vi "NI6071E.evt call DAQ Config.vi"(0 "i ref in":refnum<vi>, 2 "Client":string, 3 "Client timeout (10000)":i32=10000, 4 "NI6071E Config":T1={"device (1)"=1, "channels (0)"=[], "buffer size (1000 scans)"=1000, "[number of buffers] (1)"=1, "measurement mode structure"={"measurement mode"=0, "reserved"=0}, "input limits (no change)"=[], "coupling & input config (no change:0)"=[]} {"measurement mode structure"."measurement mode" items=["no change", "Volts", "Volts RMS", "Ohms", "Diode", "4-wire ohms", "Current", "Current RMS"]; "coupling & input config (no change:0)"."input config (no change:0)" items=["no change", "differential", "ref. single-ended", "non-ref. single-ended", "4-wire"]; "input limits (no change)"."low limit (0.0)" format="%0.2f"; "input limits (no change)"."high limit (0.0)" format="%0.2f"}, 5 "error in (no error)":errorcluster) -> (14 "i ref out":refnum<vi>, 19 "error out":errorcluster)   [LabVIEW 2014, in "NI6071E.lvlib"]
doc: "This VI asks for an event by a simple call"
uses:
  NI6071E.lvlib
  NI6071ECommand.ctl
  NI6071EConfig.ctl
  CSCore/CSSystem/CoreLib/CoreLib.string 2 byte array.vi
  CSCore/CSSystem/CoreLib/CoreLib.int 2 byte array.vi
  CSCore/BaseProcess/BaseProcess.lvlib
  CSCore/CSSystem/CoreLib/CoreLib.lvlib
panel:
  in  "NI6071E Command":T2=enum."ConfigureDAQ"
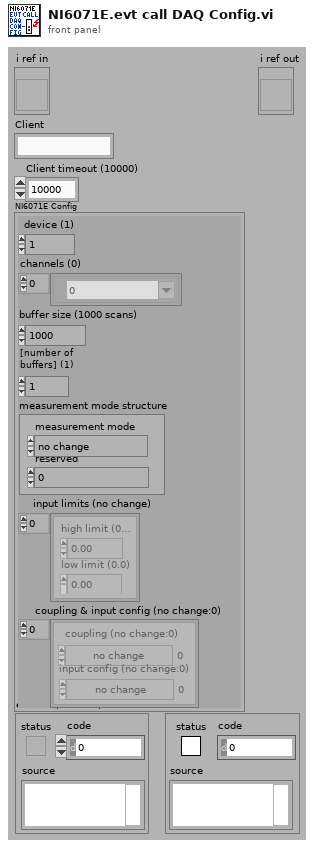
[diagram p1: front panel]
types:
  T1 = typedef "NI6071E.lvlib/NI6071EConfig.ctl" = cluster{"device (1)":i16, "channels (0)":tag[], "buffer size (1000 scans)":i32, "[number of buffers] (1)":i32, "measurement mode structure":cluster{"measurement mode":u16, "reserved":u32}, "input limits (no change)":cluster{"high limit (0.0)":sgl, "low limit (0.0)":sgl}[], "coupling & input config (no change:0)":cluster{"coupling (no change:0)":enum16{"no change", "DC", "AC", "GND", "internal ref."}, "input config (no change:0)":u16}[]}
  T2 = typedef "NI6071E.lvlib/NI6071ECommand.ctl" = enum16{"Ping", "Reset", "ConfigureDAQ", "StartDAQ", "StopDAQ", "GetDAQStatus", "ReadData", "SaveData", "CloseConnection"}
  T3 = typedef "CoreDefs.rawDataType.ctl" = i8[]
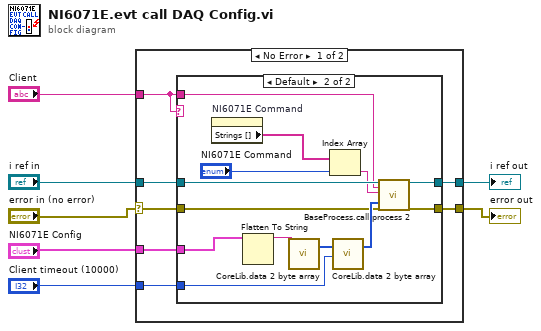
[diagram p0: block diagram]
diagram:
  n1 = case shown="No Error" "error in (no error)" {
    selector: "error in (no error)" -> [w9 w30]
    tunnel: [w14 w30] -> w7
    tunnel: "i ref in" -> [w13 w31]
    tunnel: "Client" -> [w8 _]
    tunnel: [w12 w31] -> w4
    tunnel: "NI6071E Config" -> [w11 _]
    tunnel: "Client timeout (10000)" -> [w10 _]
    frame No Error {
      n2 = case shown="Default" w8 {
        tunnel: [w15 w29] -> w14
        tunnel: w13 -> [w16 w28]
        tunnel: w8 -> [_ w27]
        tunnel: [w16 w26] -> w12
        tunnel: w11 -> [_ w20]
        tunnel: w10 -> [_ w19]
        tunnel: w9 -> [w15 w17]
        frame "N/A" {
        }
        frame Default {
          n3 = property on="NI6071E Command" class="Enum (strict)"() -> ("Strings []"=w24:string[])  [unwired: 2 in, 2 out]
          n4 = Flatten To String(anything=w20) -> (data string=w21:string)  [unwired: 3 in, 2 out]
          n5 = call-poly "CoreLib.data 2 byte array.vi"("string"=w21) -> ("byteArray out"=w22:T3)  [unwired: 18 in]
          n6 = Index Array(array=w24, index="NI6071E Command") -> (element=w23:string)
          n7 = call-poly "CoreLib.data 2 byte array.vi"("byteArray"=w22, "i32"=w19) -> ("byteArray out"=w18:T3)  [unwired: 17 in]
          n8 = call "BaseProcess.call process 2.vi"("i ref in"=w28, "Object"=w27, "Selector"=w23, "Data"=w18, "error in (no error)"=w17) -> ("i ref out"=w26:refnum<vi>, "error out"=w29:errorcluster)  [unwired: 13 in]
        }
      }
    }
    frame Error {
    }
  }
  "error out" <- w7
  "i ref out" <- w4
